vi "Keithley617_Write_GPIB_Command.vi"(6 "Execute Command?":bool=TRUE, 7 "GPIB Address String":string="27", 8 "Error In":errorcluster, 10 "Value":dbl, 11 "Command":T1="X") -> (0 "Error Out":errorcluster)   [LabVIEW 2015, in "Keithley617.lvlib"]
uses:
  Keithley617.lvlib
  Keithley617_GPIB_Commands.ctl
  <vilib>/Utility/error.llb/Error Cluster From Error Code.vi
  <vilib>/ErrorRing/Error Ring.xnode
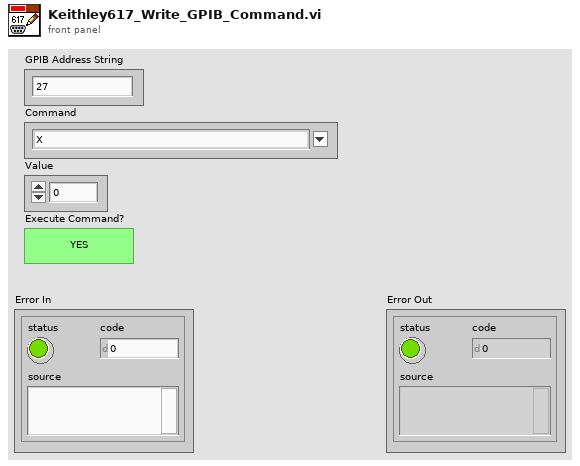
[diagram p1: front panel]
types:
  T1 = typedef "Keithley617_GPIB_Commands.ctl" = string
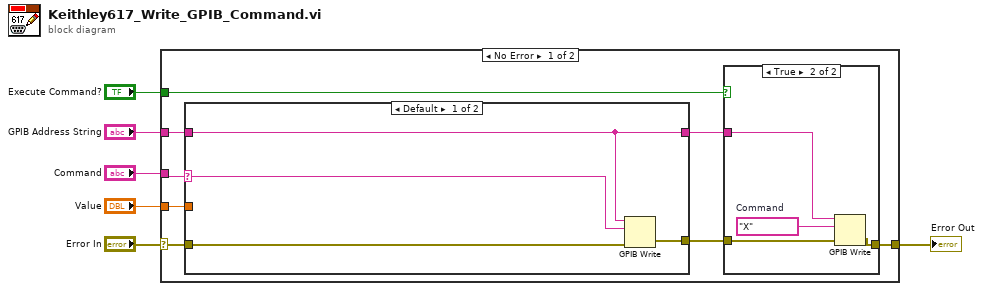
[diagram p0: block diagram]
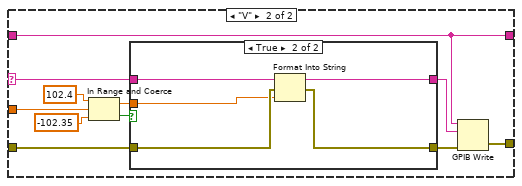
[diagram p2: hidden frame]
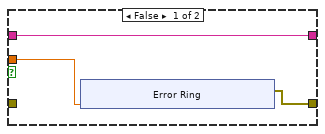
[diagram p3: hidden frame]
diagram:
  n1 = case shown="No Error" "Error In" {
    selector: "Error In" -> [w14 w50]
    tunnel: [w11 w50] -> w5
    tunnel: "GPIB Address String" -> [w13 _]
    tunnel: "Command" -> [w9 _]
    tunnel: "Execute Command?" -> [w10 _]
    tunnel: "Value" -> [w8 _]
    frame No Error {
      n2 = case shown="Default" w9 {
        selector: w9 -> [w16 w24]
        tunnel: w14 -> [w18 w22]
        tunnel: w13 -> [w15 w19]
        tunnel: [w17 w29] -> w12
        tunnel: w8 -> [_ w28]
        tunnel: [w15 w19] -> w7
        frame Default {
          n3 = GPIB Write(0:w15, 1:w16, 3:w18) -> (6:w17:errorcluster)  [unwired: 2 in, 1 out]
        }
        frame "V" {
          n4 = In Range and Coerce(upper limit=102.4, x=w28, lower limit=-102.35) -> (coerced(x)=w25:dbl, In Range?=w23:bool)
          n5 = case shown="True" w23 {
            tunnel: w25 -> [w31 w40]
            tunnel: w24 -> [w32 w44]
            tunnel: w22 -> [_ w43]
            tunnel: [w30 w42] -> w21
            tunnel: [w32 w41] -> w20
            frame False {
              n6 = xnode "Error Ring"("parameter 0"=w31) -> ("error out"=w30:errorcluster)
            }
            frame True {
              n7 = Format Into String(initial string=w44, error in=w43, w40) -> (resulting string=w41:string, error out=w42:errorcluster)  [unwired: 1 in]
            }
          }
          n8 = GPIB Write(0:w19, 1:w20, 3:w21) -> (6:w29:errorcluster)  [unwired: 2 in, 1 out]
        }
      }
      n9 = case shown="True" w10 {
        tunnel: w7 -> [_ w49]
        tunnel: w12 -> [w45 w47]
        tunnel: [w45 w46] -> w11
        frame False {
        }
        frame True {
          w48 = T1 "X"  # Command
          n10 = GPIB Write(0:w49, 1:w48, 3:w47) -> (6:w46:errorcluster)  [unwired: 2 in, 1 out]
        }
      }
    }
    frame Error {
    }
  }
  "Error Out" <- w5
